vi "ESensor.vi"() -> ()   [LabVIEW 2014]
uses:
  <vilib>/Analysis/baseanly.llb/Mean (DBL).vi
  <vilib>/DAQmx/create/channels.llb/DAQmx Create Channel (AI-Voltage-Basic).vi
  <vilib>/DAQmx/configure/timing.llb/DAQmx Timing (Sample Clock).vi
  <vilib>/DAQmx/read.llb/DAQmx Read (Analog 1D DBL 1Chan NSamp).vi
  <vilib>/Analysis/NI_AALBase.lvlib
panel:
  out "Concentration (%)":dbl format="%.4f%"
  in  "Pause chart":bool
  in  "Gain":dbl=3.31
  in  "Offset":dbl=-0.032 step=0.01 format="%_3f"
  in  "K1":dbl=-2.995 format="%#_13g"
  in  "K0":dbl=0.9054 format="%#_13g"
  out "mean (V)":dbl=0.8101309205695689 format="%.3f"
  in  "Clear Chart":bool
  out "Waveform Chart":dbl(graph)=5.598482783727609
  in  "samples per channel":i32=10
  in  "rate":dbl=100.0 format="%0.2f"
  in  "physical channels":tag="Dev2/ai23"
  in  "stop":bool
  # "by L.Andrzejewski\nlandrzej@uottawa.ca"
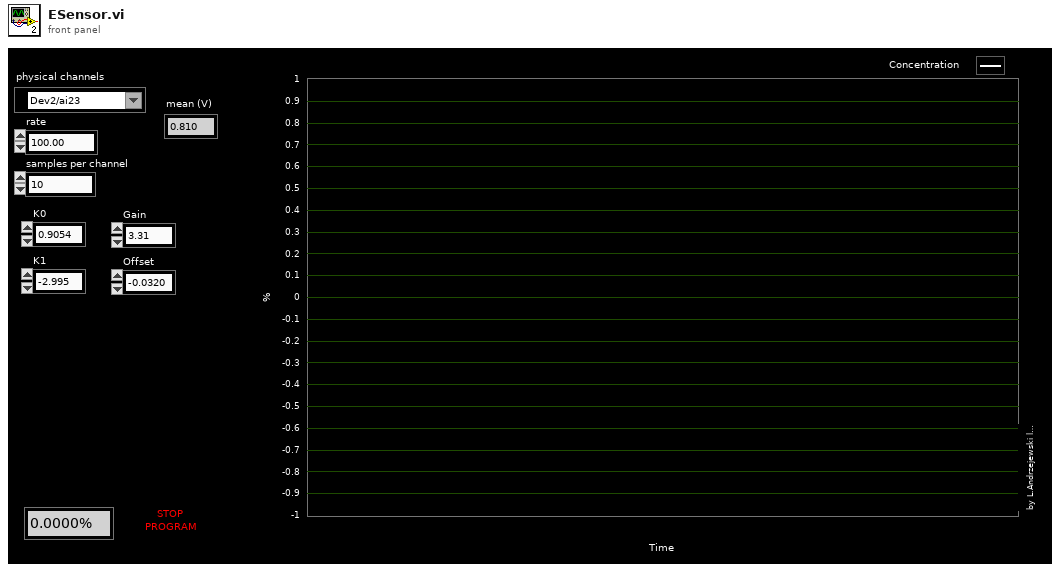
[diagram p1: front panel]
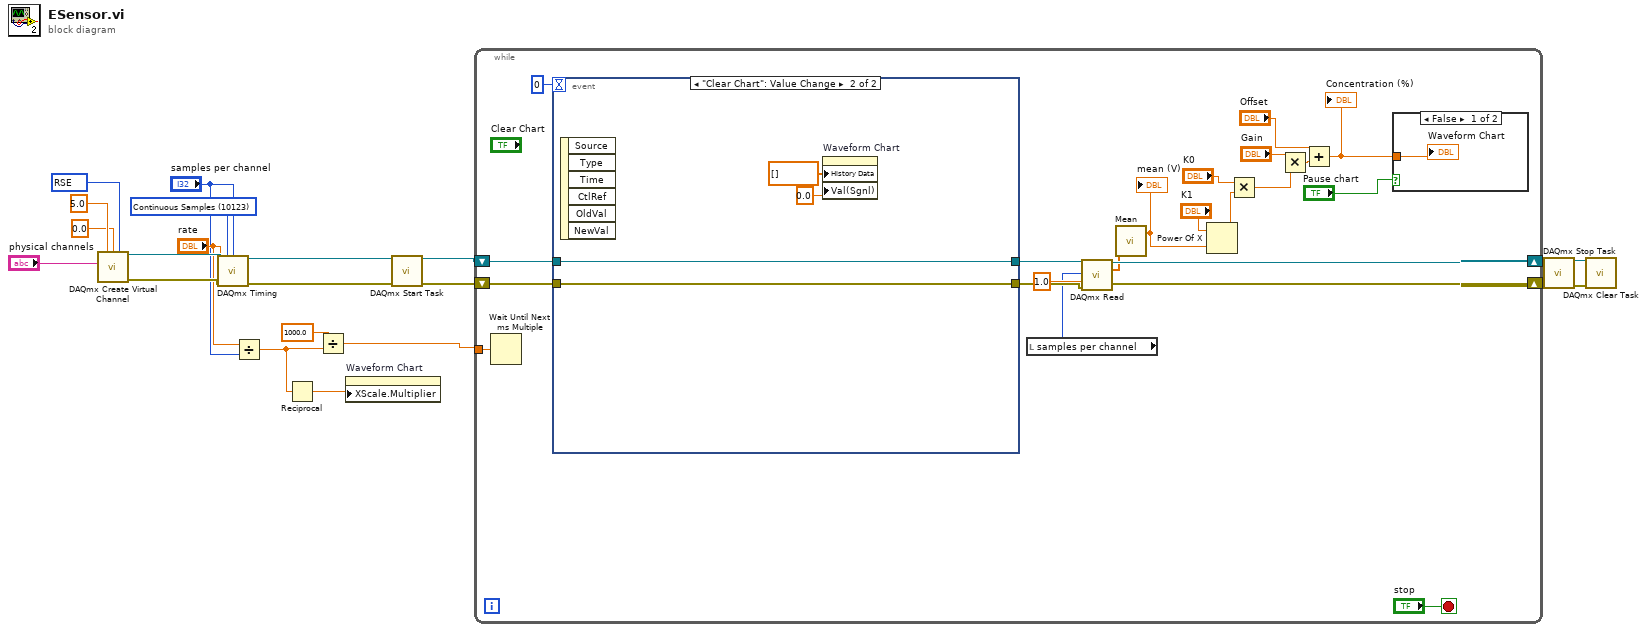
[diagram p0: block diagram]
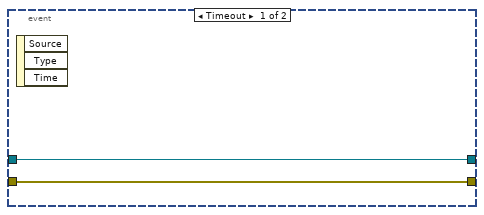
[diagram p3: hidden frame]
diagram:
  w16 = 10123 items=["Finite Samples"=10178, "Continuous Samples"=10123, "Hardware Timed Single Point"=12522] ("sample mode")
  w18 = 10083 items=["default"=-1, "RSE"=10083, "NRSE"=10078, "Differential"=10106, "Pseudodifferential"=12529] ("input terminal configuration")
  n1 = call-poly <vilib>:"DAQmx Create Virtual Channel.vi"("maximum value"=5.0, "minimum value"=0.0, "input terminal configuration"=w18, "physical channels"="physical channels") -> ("task out"=w17:refnum<k21>, "error out"=w15:errorcluster)  [unwired: 10 in]
  n2 = call-poly <vilib>:"DAQmx Timing.vi"("task/channels in"=w17, "sample mode"=w16, "samples per channel"="samples per channel", "rate"="rate", "error in"=w15) -> ("task out"=w14:refnum<k21>, "error out"=w13:errorcluster)  [unwired: 9 in]
  n3 = Divide(x="rate", y="samples per channel") -> (x/y=w1:dbl)
  n4 = Reciprocal(x=w1) -> (1/x=w2:dbl)
  n5 = Divide(x=1000.0 ("y"), y=w1) -> (x/y=w4:dbl)
  n6 = property on="Waveform Chart" class="WFChart (strict)"("XScale.Multiplier"=w2) -> ()  [unwired: 2 in, 2 out]
  n7 = call <vilib>:"DAQmx Start Task.vi"("task/channels in"=w14, "error in"=w13) -> ("task out"=w12:refnum<k21>, "error out"=w11:errorcluster)  [unwired: 12 in]
  n8 = while {
    shift-right: [w36] -> w10
    shift-left: w12 -> [w41]
    shift-right: [w35] -> w9
    shift-left: w11 -> [w40]
    tunnel: w4 -> [w29]
    stop <- "stop" stop-if-true
    n9 = Wait Until Next ms Multiple(millisecond multiple=w29) -> ()  [unwired: 1 out]
    n10 = event shown="[1] \"Clear Chart\": Value Change" {
      selector: _ -> [_ _]
      dyn-events: _ -> [_ _]
      timeout: 0 -> [_ _]
      tunnel: [w46 w50] -> w39
      tunnel: w41 -> [w46 w50]
      tunnel: [w45 w49] -> w38
      tunnel: w40 -> [w45 w49]
      event Timeout {
        n11 = event-data() -> ()  [unwired: 1 in, 3 out]
      }
      event "Clear Chart": Value Change {
        n12 = event-data() -> ()  [unwired: 1 in, 6 out]
        n13 = property on="Waveform Chart" class="WFChart (strict)"("History Data"=dbl[] [], "Val(Sgnl)"=0.0 ("Value (Signaling)")) -> ()  [unwired: 2 in, 2 out]
      }
    }
    n14 = local read "samples per channel"() -> (w30:i32)
    n15 = call-poly <vilib>:"DAQmx Read.vi"("task/channels in"=w39, "number of samples per channel"=w30, "timeout"=1.0, "error in"=w38) -> ("task out"=w36:refnum<k21>, "data"=w34:dbl[], "error out"=w35:errorcluster)  [unwired: 9 in]
    n16 = call-poly <vilib>:"Mean.vi"("X"=w34) -> ("mean"=w25:dbl)  [unwired: 1 out]
    "mean (V)" <- w25
    n17 = Power Of X(1:w25, 2:"K1") -> (0:w32:dbl)
    n18 = Multiply(x="K0", y=w32) -> (x*y=w24:dbl)
    n19 = Multiply(x="Gain", y=w24) -> (x*y=w27:dbl)
    n20 = Add(x="Offset", y=w27) -> (x+y=w23:dbl)
    "Concentration (%)" <- w23
    n21 = case shown="False" "Pause chart" {
      tunnel: w23 -> [w44 _]
      frame False {
        "Waveform Chart" <- w44
      }
      frame True {
      }
    }
  }
  n22 = call <vilib>:"DAQmx Stop Task.vi"("task/channels in"=w10, "error in"=w9) -> ("task out"=w8:refnum<k21>, "error out"=w7:errorcluster)  [unwired: 12 in]
  n23 = call <vilib>:"DAQmx Clear Task.vi"("task in"=w8, "error in"=w7) -> ()  [unwired: 13 in, 1 out]
